vi "Configure Forward Power.vi"(8 "error in (no error)":errorcluster, 10 "Pfwd, W":u16=50, 11 "HFP Gen in":refnum<class "PL HFP Generator.lvclass">) -> (0 "error out":errorcluster, 3 "HFP Gen out":refnum<class "PL HFP Generator.lvclass">)   [LabVIEW 2015, in "PL HFP Generator.lvclass"]
doc: "Configures forward power."
uses:
  PL HFP Generator.lvclass
  <vilib>/plasmapper/PL Modbus Client/PL Modbus Client.lvclass
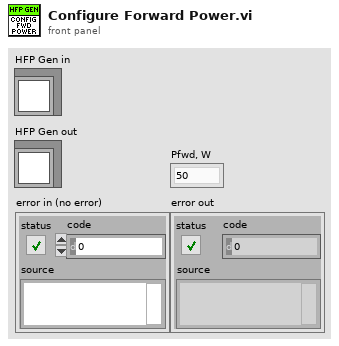
[diagram p1: front panel]
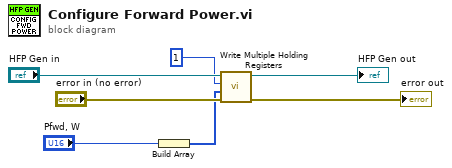
[diagram p0: block diagram]
diagram:
  n1 = Build Array("Pfwd, W") -> (w2:u16[])
  n2 = call <vilib>:"Write Multiple Holding Registers.vi"("error in (no error)"="error in (no error)", "values"=w2, "address"=u16 1, "MODBUS in"="HFP Gen in") -> ("error out"=→"error out":errorcluster, "MODBUS out"=→"HFP Gen out":refnum<class "PL HFP Generator.lvclass">)  [unwired: 6 in]
